vi "camera light.vi"() -> ()   [LabVIEW 2011]
uses:
  <vilib>/Rock Robotics/WPI/Relay/WPI_RelayValue.ctl
  <vilib>/Rock Robotics/SystemInterfaces/Typedef/FPGA_TypedefDigitalModule.ctl
  <vilib>/Rock Robotics/SystemInterfaces/DIO/FPGA_DIORelayChannel.ctl
panel:
  in  "RelayValue":T1=enum."Forward"
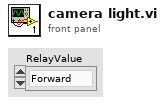
[diagram p1: front panel]
types:
  T1 = typedef "WPI_RelayValue.ctl" = enum16{"Off", "On", "Forward", "Reverse"}
  T2 = typedef "FPGA_DIORelayChannel.ctl" = enum8{"Relay 1", "Relay 2", "Relay 3", "Relay 4", "Relay 5", "Relay 6", "Relay 7", "Relay 8", "Invalid"}
  T3 = typedef "FPGA_TypedefDigitalModule.ctl" = enum16{"Digital Module 1", "Digital Module 2"}
  T4 = typedef "WPI_RelayDevRef.ctl" = cluster{"DevStatus":errorcluster, "Relay Channel":T2, "Digital Module":T3, "Relay Direction":T5}
  T5 = typedef "WPI_RelayDirection.ctl" = enum16{"Both directions", "Forward only", "Reverse only"}
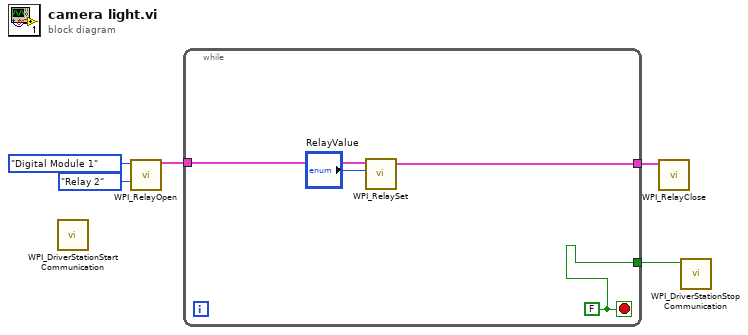
[diagram p0: block diagram]
diagram:
  n1 = call <vilib>:"WPI_DriverStationStart Communication.vi"() -> ()  [unwired: 12 in]
  n2 = call <vilib>:"WPI_RelayOpen.vi"("Relay Channel"=FPGA_DIORelayChannel."Relay 2", "Digital Module (Module 1)"=FPGA_TypedefDigitalModule."Digital Module 1") -> ("RelayDevRef"=w4:T4)  [unwired: 8 in, 1 out]
  n3 = while {
    tunnel: [w9] -> w5
    tunnel: w4 -> [w8]
    tunnel: [w6] -> w1
    stop <- w6 stop-if-true
    w6 = FALSE
    n4 = call <vilib>:"WPI_RelaySet.vi"("RelayValue"="RelayValue", "RelayDevRef"=w8) -> ("RelayDevRef"=w9:T4)  [unwired: 8 in, 1 out]
  }
  n5 = call <vilib>:"WPI_RelayClose.vi"("RelayDevRef"=w5) -> ()  [unwired: 10 in, 1 out]
  n6 = call <vilib>:"WPI_DriverStationStop Communication.vi"("StopCommunication"=w1) -> ()  [unwired: 10 in, 1 out]
